vi "EventTouch_BallPossession.vi"(6 "D bola anda":dbl=10.0, 8 "Dist Para Toque":dbl=130.0, 9 "Tol para ang posse":dbl=0.3, 10 "Dist Para posse":dbl=180.0, 11 "IA State":T1={"our_robots"=[], "enemy_robots"=[], "balls"=[], "geometry"={"line_width"=0, "field_length"=0, "field_width"=0, "boundary_width"=0, "referee_width"=0, "goal_width"=0, "goal_depth"=0, "goal_wall_width"=0, "center_circle_radius"=0, "defense_radius"=0, "defense_stretch"=0, "free_kick_from_defense_dist"=0, "penalty_spot_from_field_line_dist"=0, "penalty_line_from_spot_dist"=0}, "IA Judge"={"stage"="", "command"="", "our_goalie_id"=0.0, "enemy_goalie_id"=0.0, "command enum"=enum."Halt", "Time"=enum."Azul"}, "Received Timestamp"=timestamp(0 s since 1904-01-01), "Events"={"Touch"=FALSE, "Ball out"=FALSE, "id touch"=0.0, "Ball out of \nVision"=FALSE, "Ball inside \nGoalie area"=FALSE, "Robot not responding"=FALSE, "Robots responding status"=[1.0, 1.0, 1.0, 1.0, 1.0, 1.0], "Enemy Ball \nPossession"=FALSE, "Pass State"=FALSE, "id end of pass"=0.0, "Kick"=FALSE, "Id ini Possession"=0.0, "Ball Possesion"=FALSE, "Id Possesion"=0.0}}) -> (0 "id touch":dbl, 1 "Toque":bool, 2 "id ini possesion":dbl, 3 "Posse inimigo":bool, 5 "id possesion":dbl, 7 "Posse nossa":bool)   [LabVIEW 2017]
uses:
  Core/AI Input.ctl
  Core/AI Robot.ctl
  Intel/Functions Enum.ctl
  Intel/AttackerStates.ctl
  Path Planning/RRT/PathDests.ctl
  Path Planning/RRT/PathDest.ctl
  Core/AI Ball.ctl
  Core/Field Size.ctl
  Core/AI Judge.ctl
  Intel/Command Enum.ctl
  Events.ctl
  <vilib>/Analysis/coordinate.llb/Wrap Angle (scalar).vi
  <vilib>/Analysis/_algsub.llb/Real Vector Norm.vi
  <vilib>/Analysis/NI_AAL_Angle.lvlib
  <vilib>/Analysis/NI_AALPro.lvlib
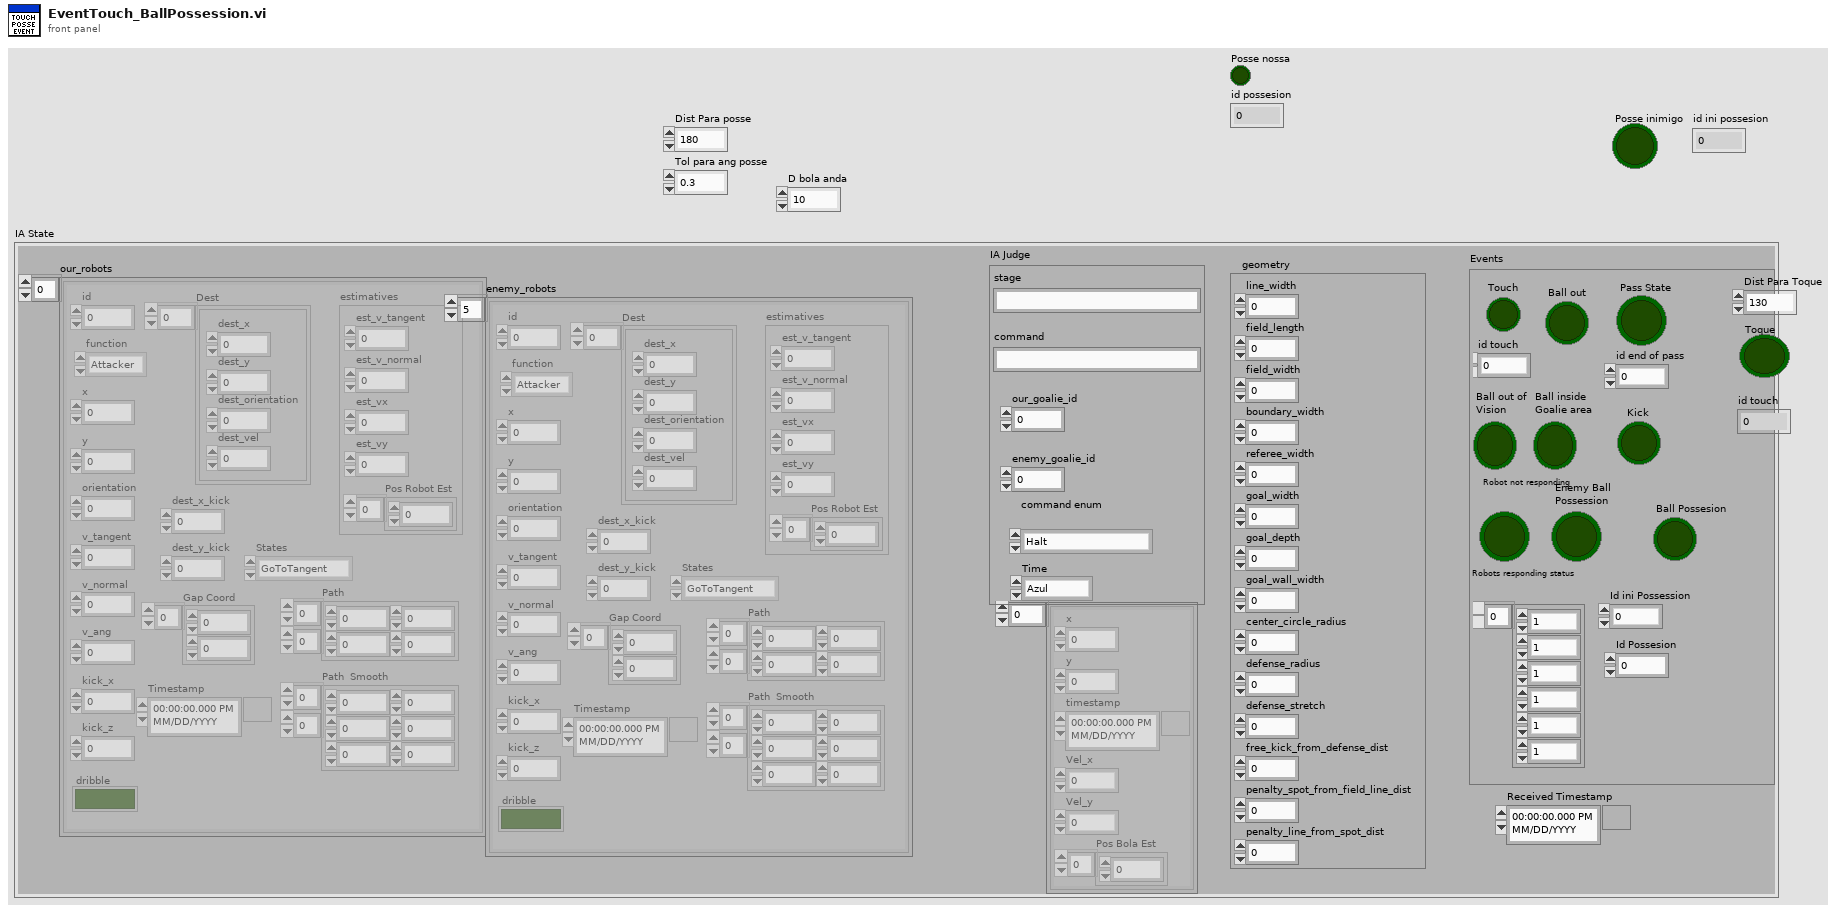
[diagram p1: front panel]
types:
  T1 = typedef "AI Input.ctl" = cluster{"our_robots":T2[], "enemy_robots":T2[], "balls":T7[], "geometry":T8, "IA Judge":T9, "Received Timestamp":timestamp, "Events":T11}
  T2 = typedef "AI Robot.ctl" = cluster{"id":u32, "function":T3, "x":dbl, "y":dbl, "orientation":dbl, "v_tangent":dbl, "v_normal":dbl, "v_ang":dbl, "kick_x":dbl, "kick_z":dbl, "dribble":bool, "Timestamp":timestamp, "estimatives":cluster{"est_v_tangent":dbl, "est_v_normal":dbl, "est_vx":dbl, "est_vy":dbl, "Pos Robot Est":dbl[]}, "dest_x_kick":dbl, "dest_y_kick":dbl, "Gap Coord":dbl[], "States":T4, "Path ":dbl[][], "Path  Smooth":dbl[][], "Dest":T5}
  T3 = typedef "Functions Enum.ctl" = enum16{"Attacker", "Goalie", "Defender", "Striker", "Goto 0", "Dummy", "Kicker", "ZigZag"}
  T4 = typedef "AttackerStates.ctl" = enum16{"Pass", "GoToTangent", "BallGetting", "GoToKick", ""}
  T5 = typedef "PathDests.ctl" = T6[]
  T6 = typedef "PathDest.ctl" = cluster{"dest_x":dbl, "dest_y":dbl, "dest_orientation":dbl, "dest_vel":dbl}
  T7 = typedef "AI Ball.ctl" = cluster{"x":dbl, "y":dbl, "timestamp":timestamp, "Vel_x":dbl, "Vel_y":dbl, "Pos Bola Est":dbl[]}
  T8 = typedef "Field Size.ctl" = cluster{"line_width":u32, "field_length":u32, "field_width":u32, "boundary_width":u32, "referee_width":u32, "goal_width":u32, "goal_depth":u32, "goal_wall_width":u32, "center_circle_radius":u32, "defense_radius":u32, "defense_stretch":u32, "free_kick_from_defense_dist":u32, "penalty_spot_from_field_line_dist":u32, "penalty_line_from_spot_dist":u32}
  T9 = typedef "AI Judge.ctl" = cluster{"stage":string, "command":string, "our_goalie_id":dbl, "enemy_goalie_id":dbl, "command enum":T10, "Time":enum16{"Azul", "Amarelo"}}
  T10 = typedef "Command Enum.ctl" = enum16{"Halt", "Stop", "Force Start", "PKA Normal Start", "Prepare Kickoff Ally", "PKE Normal Start", "Prepare Kickoff Enemy", "Prepare Penalty Ally", "PPA Normal Start", "Prepare Penalty Enemy", "PPE Normal Start", "Direct Free Enemy", "Direct Free Ally", "Indirect Free Enemy", "Indirect Free Ally", "Timeout Enemy", "Timeout Ally", "Goal Enemy", "Goal Ally", "Ball Placement Enemy", "Ball Placement Ally", "Normal Half Time", "Extra Time Break", "Extra Half Time", "None", "Post Game"}
  T11 = typedef "Events.ctl" = cluster{"Touch":bool, "Ball out":bool, "id touch":dbl, "Ball out of \nVision":bool, "Ball inside \nGoalie area":bool, "Robot not responding":bool, "Robots responding status":dbl[], "Enemy Ball \nPossession":bool, "Pass State":bool, "id end of pass":dbl, "Kick":bool, "Id ini Possession":dbl, "Ball Possesion":bool, "Id Possesion":dbl}
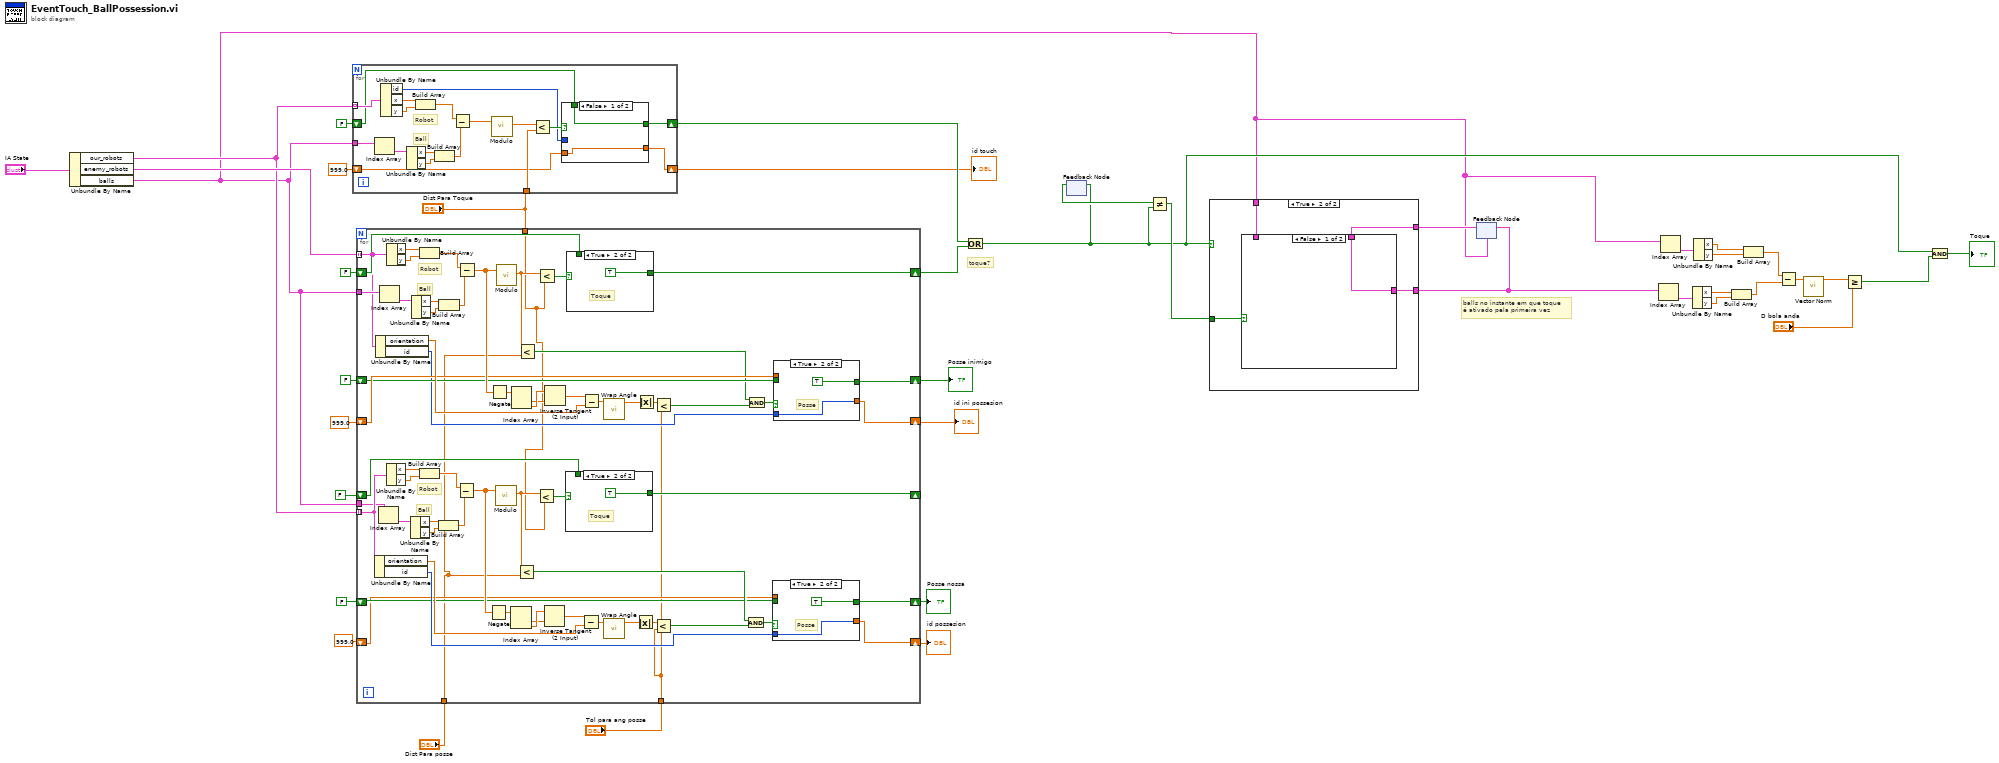
[diagram p0: block diagram]
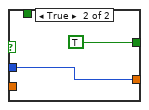
[diagram p8: hidden frame]
diagram:
  # "balls no instante em que toque\né ativado pela primeira vez"
  # "toque?"
  n1 = Unbundle By Name("IA State") -> ("our_robots"=w23:T2[], "enemy_robots"=w37:T2[], "balls"=w1:T7[])
  n2 = for {
    tunnel: w23 -> [w54] mode=indexing
    tunnel: w1 -> [w58]
    shift-right: [w46] -> w38
    shift-left: FALSE -> [w45]
    tunnel: "Dist Para Toque" -> [w44]
    shift-right: [w43] -> w34
    shift-left: 999.0 ("id") -> [w41]
    # "Ball"
    # "Robot"
    n3 = Index Array(array=w58) -> (element=w57:T7)  [unwired: 1 in]
    n4 = Unbundle By Name(w54) -> ("id"=w42:u32, "x"=w53:dbl, "y"=w52:dbl)
    n5 = Unbundle By Name(w57) -> ("x"=w56:dbl, "y"=w55:dbl)
    n6 = Build Array(w53, w52) -> (w51:dbl[])
    n7 = Build Array(w56, w55) -> (w50:dbl[])
    n8 = Subtract(x=w51, y=w50) -> (x-y=w49:dbl[])
    n9 = call "Modulo.vi"("2D vector"=w49) -> ("Modulo"=w47:dbl)  [unwired: 10 in]
    n10 = Less?(x=w47, y=w44) -> (x < y?=w48:bool)
    n11 = case shown="False" w48 {
      tunnel: [w60 TRUE] -> w46
      tunnel: w45 -> [w60 _]
      tunnel: [w59 w61] -> w43
      tunnel: w42 -> [_ w61]
      tunnel: w41 -> [w59 _]
      frame False {
      }
      frame True {
      }
    }
  }
  "id touch" <- w34
  n12 = for {
    tunnel: w37 -> [w114] mode=indexing
    tunnel: w1 -> [w125]
    shift-right: [w116] -> w36
    shift-left: FALSE -> [w115]
    tunnel: "Dist Para Toque" -> [w65]
    tunnel: "Tol para ang posse" -> [w63]
    shift-right: [w97] -> w27
    shift-left: 999.0 -> [w102]
    tunnel: "Dist Para posse" -> [w64]
    shift-right: [w101] -> w28
    shift-left: FALSE -> [w100]
    shift-right: [w72] -> _
    shift-left: FALSE -> [w73]
    shift-right: [w68] -> w22
    shift-left: FALSE -> [w71]
    shift-right: [w69] -> w21
    shift-left: 999.0 -> [w70]
    tunnel: w23 -> [w67] mode=indexing
    tunnel: w1 -> [w66]
    # "Ball"
    # "Robot"
    # "Ball"
    # "Robot"
    n13 = Unbundle By Name(w67) -> ("orientation"=w79:dbl, "id"=w74:u32)
    n14 = Unbundle By Name(w114) -> ("orientation"=w105:dbl, "id"=w96:u32)
    n15 = Index Array(array=w66) -> (element=w95:T7)  [unwired: 1 in]
    n16 = Index Array(array=w125) -> (element=w124:T7)  [unwired: 1 in]
    n17 = Unbundle By Name(w67) -> ("x"=w92:dbl, "y"=w91:dbl)
    n18 = Unbundle By Name(w114) -> ("x"=w121:dbl, "y"=w120:dbl)
    n19 = Unbundle By Name(w95) -> ("x"=w94:dbl, "y"=w93:dbl)
    n20 = Unbundle By Name(w124) -> ("x"=w123:dbl, "y"=w122:dbl)
    n21 = Build Array(w92, w91) -> (w90:dbl[])
    n22 = Build Array(w121, w120) -> (w119:dbl[])
    n23 = Build Array(w94, w93) -> (w89:dbl[])
    n24 = Build Array(w123, w122) -> (w118:dbl[])
    n25 = Subtract(x=w90, y=w89) -> (x-y=w80:dbl[])
    n26 = Subtract(x=w119, y=w118) -> (x-y=w106:dbl[])
    n27 = Negate(x=w80) -> (-x=w87:dbl[])
    n28 = Negate(x=w106) -> (-x=w113:dbl[])
    n29 = call "Modulo.vi"("2D vector"=w80) -> ("Modulo"=w78:dbl)  [unwired: 10 in]
    n30 = call "Modulo.vi"("2D vector"=w106) -> ("Modulo"=w104:dbl)  [unwired: 10 in]
    n31 = Index Array(array=w87) -> (element #1=w85:dbl, element #2=w86:dbl)  [unwired: 2 in]
    n32 = Index Array(array=w113) -> (element #1=w111:dbl, element #2=w112:dbl)  [unwired: 2 in]
    n33 = Less?(x=w78, y=w64) -> (x < y?=w75:bool)
    n34 = Less?(x=w104, y=w64) -> (x < y?=w98:bool)
    n35 = Less?(x=w78, y=w65) -> (x < y?=w88:bool)
    n36 = Less?(x=w104, y=w65) -> (x < y?=w117:bool)
    n37 = Inverse Tangent (2 Input)(1:w85, 2:w86) -> (0:w84:dbl)
    n38 = Inverse Tangent (2 Input)(1:w111, 2:w112) -> (0:w110:dbl)
    n39 = case shown="True" w88 {
      tunnel: [w130 TRUE] -> w72
      tunnel: w73 -> [w130 _]
      frame False {
        # "Sem toque"
      }
      frame True {
        # "Toque"
      }
    }
    n40 = case shown="True" w117 {
      tunnel: [w136 TRUE] -> w116
      tunnel: w115 -> [w136 _]
      frame False {
        # "Sem toque"
      }
      frame True {
        # "Toque"
      }
    }
    n41 = Subtract(x=w84, y=w79) -> (x-y=w83:dbl)
    n42 = Subtract(x=w110, y=w105) -> (x-y=w109:dbl)
    n43 = call-poly <vilib>:"Wrap Angle.vi"("angle in"=w109) -> ("angle out"=w107:dbl)  [unwired: 9 in, 1 out]
    n44 = call-poly <vilib>:"Wrap Angle.vi"("angle in"=w83) -> ("angle out"=w81:dbl)  [unwired: 9 in, 1 out]
    n45 = Absolute Value(x=w81) -> (abs(x)=w82:dbl)
    n46 = Absolute Value(x=w107) -> (abs(x)=w108:dbl)
    n47 = Less?(x=w82, y=w63) -> (x < y?=w76:bool)
    n48 = Less?(x=w108, y=w63) -> (x < y?=w99:bool)
    n49 = And(x=w75, y=w76) -> (x .and. y?=w77:bool)
    n50 = And(x=w98, y=w99) -> (x .and. y?=w103:bool)
    n51 = case shown="True" w77 {
      tunnel: [w126 TRUE] -> w68
      tunnel: w74 -> [_ w128]
      tunnel: [w127 w128] -> w69
      tunnel: w70 -> [w127 _]
      tunnel: w71 -> [w126 _]
      frame False {
        # "Sem toque"
      }
      frame True {
        # "Posse"
      }
    }
    n52 = case shown="True" w103 {
      tunnel: [w132 TRUE] -> w101
      tunnel: w96 -> [_ w134]
      tunnel: [w133 w134] -> w97
      tunnel: w102 -> [w133 _]
      tunnel: w100 -> [w132 _]
      frame False {
        # "Sem toque"
      }
      frame True {
        # "Posse"
      }
    }
  }
  "Posse inimigo" <- w28
  "id ini possesion" <- w27
  "Posse nossa" <- w22
  "id possesion" <- w21
  n53 = Or(x=w38, y=w36) -> (x .or. y?=w3:bool)
  n54 = feedback-in #1(w3) -> ()
  n55 = feedback #1() -> (w19:bool)  [unwired: 1 in]
  n56 = Not Equal?(x=w19, y=w3) -> (x != y?=w18:bool)
  n57 = feedback #2(w1) -> (w17:T7[])
  n58 = case shown="True" w3 {
    tunnel: w1 -> [_ w139]
    tunnel: [w138 w141] -> w16
    tunnel: w18 -> [_ w142]
    tunnel: w17 -> [w138 w140]
    frame False {
    }
    frame True {
      n59 = case shown="False" w142 {
        tunnel: [w143 w144] -> w141
        tunnel: w140 -> [w143 _]
        tunnel: w139 -> [_ w144]
        frame False {
        }
        frame True {
        }
      }
    }
  }
  n60 = feedback-in #2(w16) -> ()
  n61 = Index Array(array=w16) -> (element=w15:T7)  [unwired: 1 in]
  n62 = Index Array(array=w1) -> (element=w14:T7)  [unwired: 1 in]
  n63 = Unbundle By Name(w15) -> ("x"=w13:dbl, "y"=w12:dbl)
  n64 = Unbundle By Name(w14) -> ("x"=w11:dbl, "y"=w10:dbl)
  n65 = Build Array(w13, w12) -> (w8:dbl[])
  n66 = Build Array(w11, w10) -> (w9:dbl[])
  n67 = Subtract(x=w9, y=w8) -> (x-y=w7:dbl[])
  n68 = call-poly <vilib>:"Vector Norm.vi"("Input Vector"=w7) -> ("norm"=w6:dbl)  [unwired: 9 in, 1 out]
  n69 = Greater Or Equal?(x=w6, y="D bola anda") -> (x >= y?=w4:bool)
  n70 = And(x=w3, y=w4) -> (x .and. y?=→"Toque":bool)
